vi "Register for Printf Event.vi"(8 "error in (no error)":errorcluster, 11 "Event Registration Refnum in":refnum<event-registration>) -> (0 "error out":errorcluster, 2 "Verbose Level":i32, 3 "Event Registration Refnum out":refnum<event-registration>)   [LabVIEW 2013]
uses:
  LV_Printf Core.lvclass
  Messages/General/LV_Printf Msg.lvclass
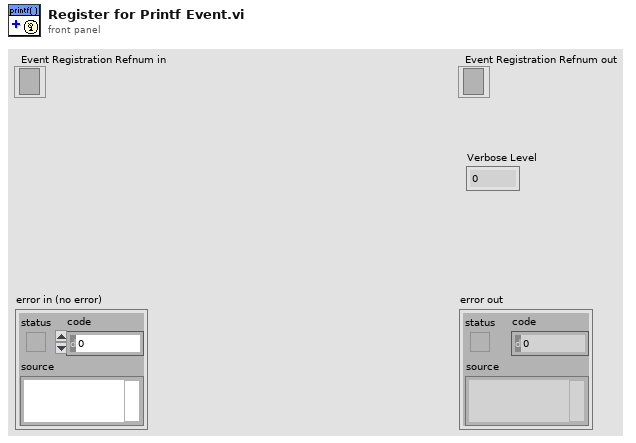
[diagram p1: front panel]
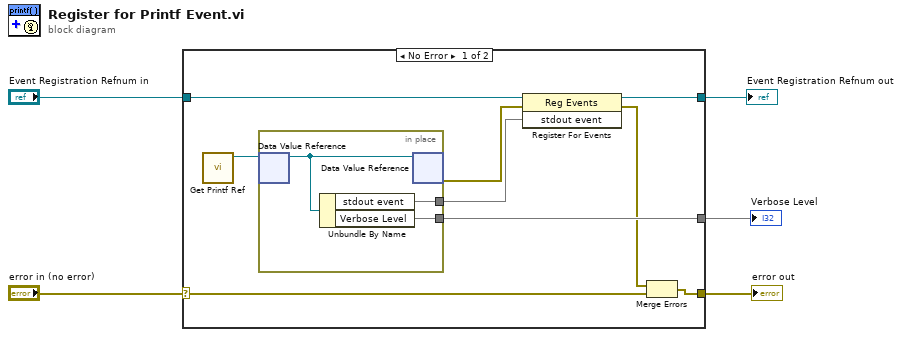
[diagram p0: block diagram]
diagram:
  n1 = case shown="No Error" "error in (no error)" {
    selector: "error in (no error)" -> [w7 w18]
    tunnel: "Event Registration Refnum in" -> [w14 w19]
    tunnel: [w13 w19] -> w4
    tunnel: [w9 _] -> w3
    tunnel: [w8 w18] -> w2
    frame No Error {
      n2 = call "Get Printf Ref.vi"() -> ("Printf DVR"=w12:refnum<data-value>)  [unwired: 11 in]
      n3 = in-place {
        in-place-border: [w16] -> w10
        in-place-border: [w15] -> w9
        n4 = in-place-dvr #1(w12) -> (w17:refnum<class "LV_Printf Core.lvclass">)  [unwired: 1 out]
        n5 = Unbundle By Name(w17) -> ("stdout event"=w16, "Verbose Level"=w15)
        n6 = in-place-dvr #1(w17) -> (w11:errorcluster)  [unwired: 1 out]
      }
      n7 = register-events(reference=w14, error in=w11, w10) -> (reference out=w13:refnum<event-registration>, error out=w6:errorcluster)
      n8 = Merge Errors(w6, w7) -> (w8:errorcluster)
    }
    frame Error {
    }
  }
  "error out" <- w2
  "Event Registration Refnum out" <- w4
  "Verbose Level" <- w3
